vi "Charging_Stop Charging.vi"(8 "error in (no error)":errorcluster, 10 "waveform handle (0)":i32, 11 "logical name (\"SampleFGen\")":refnum<k15> caption="instrument handle") -> (0 "error out":errorcluster)   [LabVIEW 2010]
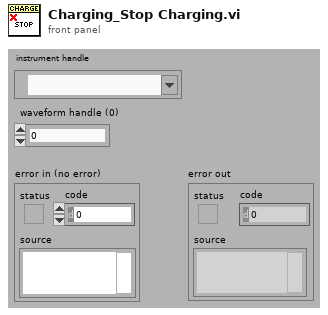
[diagram p1: front panel]
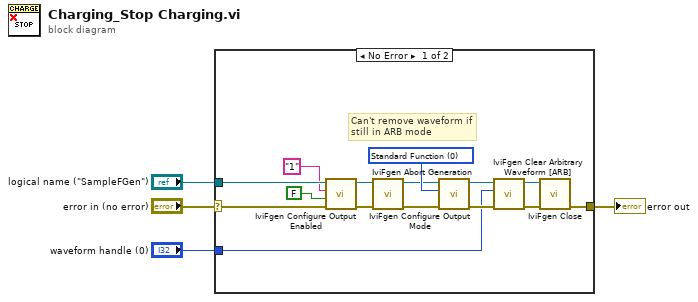
[diagram p0: block diagram]
diagram:
  n1 = case shown="No Error" "error in (no error)" {
    selector: "error in (no error)" -> [w10 w20]
    tunnel: [w8 w20] -> w3
    tunnel: "logical name (\"SampleFGen\")" -> [w11 _]
    tunnel: "waveform handle (0)" -> [w5 _]
    frame No Error {
      w16 = 0 items=["Standard Function", "Arbitrary Waveform", "Arbitrary Sequence"] ("output mode (Standard Function)")
      # "Can't remove waveform if\nstill in ARB mode"
      n2 = call <vilib>:"IviFgen Configure Output Enabled.vi"("error in (no error)"=w10, "channel enabled (True)"=FALSE, "channel name (\"CHANNEL1\")"="1" ("channel name (\"CHANNEL1\")"), "instrument handle"=w11) -> ("error out"=w19:errorcluster, "instrument handle out"=w17:refnum<k15>)  [unwired: 6 in]
      n3 = call <vilib>:"IviFgen Abort Generation.vi"("error in (no error)"=w19, "instrument handle"=w17) -> ("error out"=w14:errorcluster, "instrument handle out"=w15:refnum<k15>)  [unwired: 8 in]
      n4 = call <vilib>:"IviFgen Configure Output Mode.vi"("error in (no error)"=w14, "output mode (Standard Function)"=w16, "instrument handle"=w15) -> ("error out"=w12:errorcluster, "instrument handle out"=w13:refnum<k15>)  [unwired: 7 in]
      n5 = call <vilib>:"IviFgen Clear Arbitrary Waveform [ARB].vi"("error in (no error)"=w12, "waveform handle (0)"=w5, "instrument handle"=w13) -> ("error out"=w9:errorcluster, "instrument handle out"=w7:refnum<k15>)  [unwired: 7 in]
      n6 = call <vilib>:"IviFgen Close.vi"("error in (no error)"=w9, "instrument handle"=w7) -> ("error out"=w8:errorcluster)  [unwired: 9 in]
    }
    frame Error {
    }
  }
  "error out" <- w3
